vi "Projection_Pursuit.vi"() -> ()   [LabVIEW 2014]
uses:
  <vilib>/Analysis/baseanly.llb/A x Vector.vi
  <vilib>/Analysis/baseanly.llb/Real A x B.vi
  <vilib>/Analysis/Matrix/Numeric/Absolute Value/Absolute Value - RM.vi
  <vilib>/Analysis/NI_AALBase.lvlib
  <vilib>/Analysis/Matrix/NI_Matrix.lvlib
panel:
  in  "Input Data (X)":dbl[][](array[numeric]) format="%0.3f"
  out "W":dbl[](array[numeric])
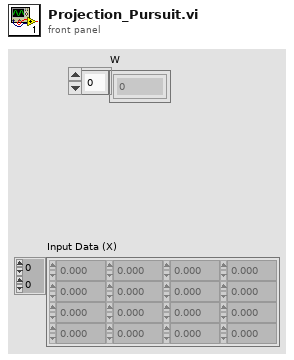
[diagram p1: front panel]
types:
  T1 = typedef "NI_Matrix.lvlib/RealMatrix.ctl" = dbl[][]
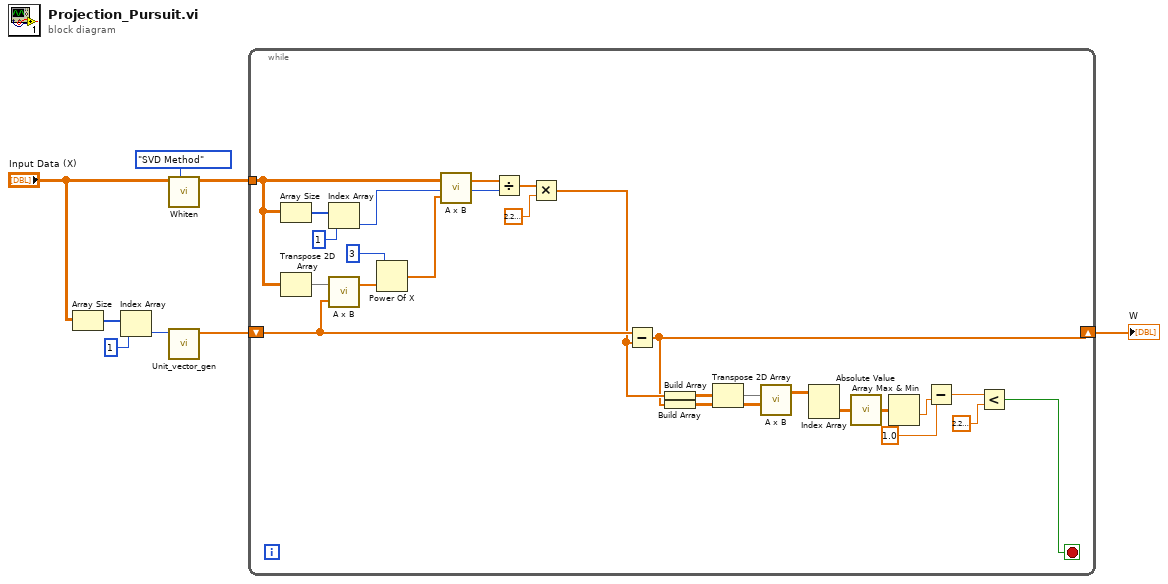
[diagram p0: block diagram]
diagram:
  n1 = Array Size(array="Input Data (X)") -> (size(s)=w6:i32[])
  n2 = Index Array(array=w6, index=1) -> (element=w4:i32)
  n3 = call "Whiten.vi"("Opt"=enum16{"SVD Method", "Inverse Method"}."SVD Method", "X (Data Matrix)"="Input Data (X)") -> ("newVector"=w8:T1)  [unwired: 7 in, 2 out]
  n4 = call "Unit_vector_gen.vi"("Length"=w4) -> ("Unit_length_Vector"=w7:dbl[])  [unwired: 10 in]
  n5 = while {
    tunnel: w8 -> [w27]
    shift-right: [w20] -> w2
    shift-left: w7 -> [w22]
    stop <- w9 stop-if-true
    n6 = Array Size(array=w27) -> (size(s)=w29:i32[])
    n7 = Transpose 2D Array(2D array=w27) -> (transposed array=w33:T1)
    n8 = Index Array(array=w29, index=1) -> (element=w25:i32)
    n9 = call-poly <vilib>:"A x B.vi"("Vector"=w22, "A"=w33) -> ("A x Vector"=w32:dbl[])  [unwired: 1 out]
    n10 = Power Of X(1:w32, 2:3) -> (0:w30:dbl[])
    n11 = call-poly <vilib>:"A x B.vi"("Vector"=w30, "A"=w27) -> ("A x Vector"=w26:dbl[])  [unwired: 1 out]
    n12 = Divide(x=w26, y=w25) -> (x/y=w23:dbl[])
    n13 = Multiply(x=w23, y=2.220446049250313e-16) -> (x*y=w21:dbl[])
    n14 = Subtract(x=w22, y=w21) -> (x-y=w20:dbl[])
    n15 = Build Array(w21) -> (w19:dbl[][])
    n16 = Build Array(w20) -> (w17:dbl[][])
    n17 = Transpose 2D Array(2D array=w19) -> (transposed array=w18:dbl[][])
    n18 = call-poly <vilib>:"A x B.vi"("B"=w17, "A"=w18) -> ("A x B"=w16:T1)  [unwired: 1 out]
    n19 = Index Array(array=w16) -> (element=w15:T1)  [unwired: 2 in]
    n20 = call-poly <vilib>:"Absolute Value.vi"("Real Matrix A"=w15) -> ("|A|"=w14:T1)
    n21 = Array Max & Min(array=w14) -> (min value=w13:dbl)  [unwired: 3 out]
    n22 = Subtract(x=1.0, y=w13) -> (x-y=w10:dbl)
    n23 = Less?(x=w10, y=2.220446049250313e-16) -> (x < y?=w9:bool)
  }
  "W" <- w2
